vi "InitPort.vi"(6 "timeout":dbl, 8 "error in (no error)":errorcluster, 9 "Baud":u32=115200, 10 "Port":string, 11 "Python":T1) -> (0 "error out":errorcluster, 2 "Console":string, 3 "Python out":T1)   [LabVIEW 2020]
uses:
  PythonCtrl.ctl
  Processors.ctl
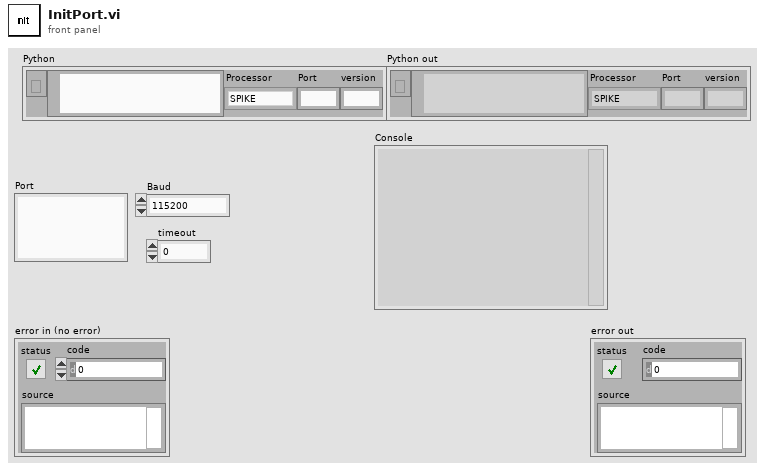
[diagram p1: front panel]
types:
  T1 = typedef "PythonCtrl.ctl" = cluster{"session":refnum<k35>, "PyPath":path, "Processor":T2, "Port":string, "version":string}
  T2 = typedef "Processors.ctl" = enum16{"SPIKE", "Pi", "Pi_ssh", "OpenMV", "Dunio"}
  T3 = cluster{"IP Address":string, "Username":string, "password":string}
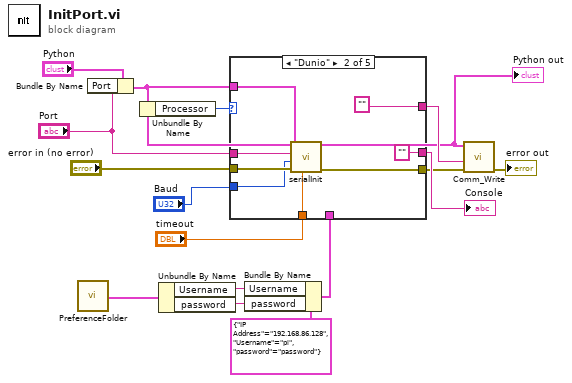
[diagram p0: block diagram]
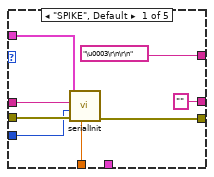
[diagram p2: hidden frame]
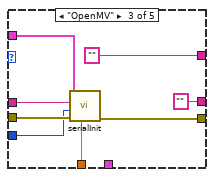
[diagram p3: hidden frame]
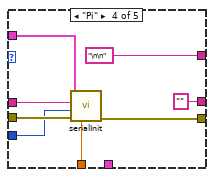
[diagram p4: hidden frame]
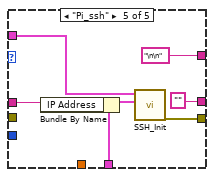
[diagram p5: hidden frame]
diagram:
  n1 = call "PreferenceFolder.vi"() -> ("Pi credentials"=w10:cluster{"Username":string, "password":string})  [unwired: 6 in, 5 out]
  n2 = Bundle By Name(cluster="Python", "Port"="Port") -> (w1:T1)
  "Python out" <- w1
  n3 = Unbundle By Name(w1) -> ("Processor"=w16:T2)
  n4 = Unbundle By Name(w10) -> ("Username"=w8:string, "password"=w9:string)
  n5 = Bundle By Name(cluster=T3 {"IP Address"="192.168.86.128", "Username"="pi", "password"="password"} ("Raspberry Pi"), "Username"=w8, "password"=w9) -> (w11:T3)
  n6 = case shown="\"Dunio\"" w16 {
    tunnel: ["\u0003\r\n\r\n" ("function name") "" ("function name") "" ("function name") "\n\n" ("function name") "\n\n" ("function name")] -> w7
    tunnel: "error in (no error)" -> [w23 w31 w39 w47 _]
    tunnel: "Port" -> [w22 w30 w38 w46 w50]
    tunnel: w1 -> [w21 w29 w37 w45 w54]
    tunnel: [w20 w28 w36 w44 w53] -> w5
    tunnel: w11 -> [_ _ _ _ w52]
    tunnel: "Baud" -> [w19 w27 w35 w43 _]
    tunnel: "timeout" -> [w18 w26 w34 w42 _]
    tunnel: ["" ("function name") "" ("function name") "" ("function name") "" ("function name") "" ("function name")] -> w6
    frame "SPIKE", Default {
      n7 = call "serialInit.vi"("timeout"=w18, "error in (no error)"=w23, "Baud"=w19, "Port"=w22, "Python"=w21) -> ("error out"=w20:errorcluster)  [unwired: 4 in, 2 out]
    }
    frame "Dunio" {
      n8 = call "serialInit.vi"("timeout"=w26, "error in (no error)"=w31, "Baud"=w27, "Port"=w30, "Python"=w29) -> ("error out"=w28:errorcluster)  [unwired: 4 in, 2 out]
    }
    frame "OpenMV" {
      n9 = call "serialInit.vi"("timeout"=w34, "error in (no error)"=w39, "Baud"=w35, "Port"=w38, "Python"=w37) -> ("error out"=w36:errorcluster)  [unwired: 4 in, 2 out]
    }
    frame "Pi" {
      n10 = call "serialInit.vi"("timeout"=w42, "error in (no error)"=w47, "Baud"=w43, "Port"=w46, "Python"=w45) -> ("error out"=w44:errorcluster)  [unwired: 4 in, 2 out]
    }
    frame "Pi_ssh" {
      n11 = Bundle By Name(cluster=w52, "IP Address"=w50) -> (w51:T3)
      n12 = call "SSH_Init.vi"("Raspberry Pi"=w51, "Python in"=w54) -> ("error out"=w53:errorcluster)  [unwired: 7 in, 2 out]
    }
  }
  "Console" <- w6
  n13 = call "Comm_Write.vi"("error in (no error)"=w5, "Text to write"=w7, "Python"=w1) -> ("error out"=→"error out":errorcluster)  [unwired: 8 in]
